vi "浮点转整形CDAB.vi"(11 "浮点":sgl[](array[numeric])) -> (3 "整形CDAB":u16[](array[numeric]) format="%04xH")   [LabVIEW 2016, in "流量计集成.lvlib" / "斯坦道功率测流.lvlib"]
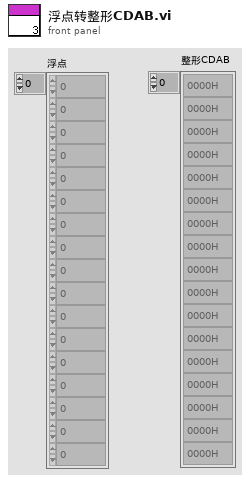
[diagram p1: front panel]
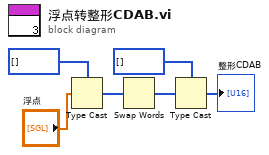
[diagram p0: block diagram]
diagram:
  n1 = Type Cast(type=u32[] [], x="浮点") -> (*(type *) &x=w4:u32[])
  n2 = Swap Words(1:w4) -> (0:w3:u32[])
  n3 = Type Cast(type=u16[] [], x=w3) -> (*(type *) &x=→"整形CDAB":u16[])
